vi "terminatePassPlay.vi"(8 "error in (no error)":errorcluster, 11 "Game in":refnum<class "Game.lvclass">) -> (0 "error out":errorcluster, 2 "terminate":bool, 3 "Game out":refnum<class "Game.lvclass">)   [LabVIEW 2018, in "Game.lvclass"]
uses:
  Game.lvclass
  Game.lvclass/Game.ctl
  Events_class/Events.lvclass/Events.ctl
  Read EventsRef.vi
  Events_class/Read ball_out.vi
  Events_class/Read touch.vi
  Events_class/Read id_touch.vi
  Events_class/Events.lvclass
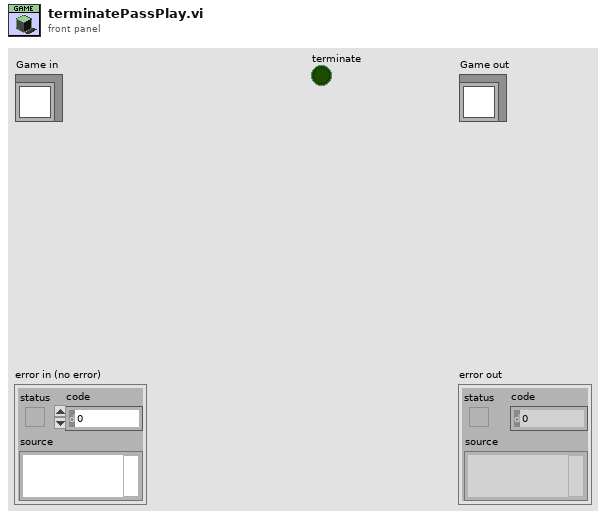
[diagram p1: front panel]
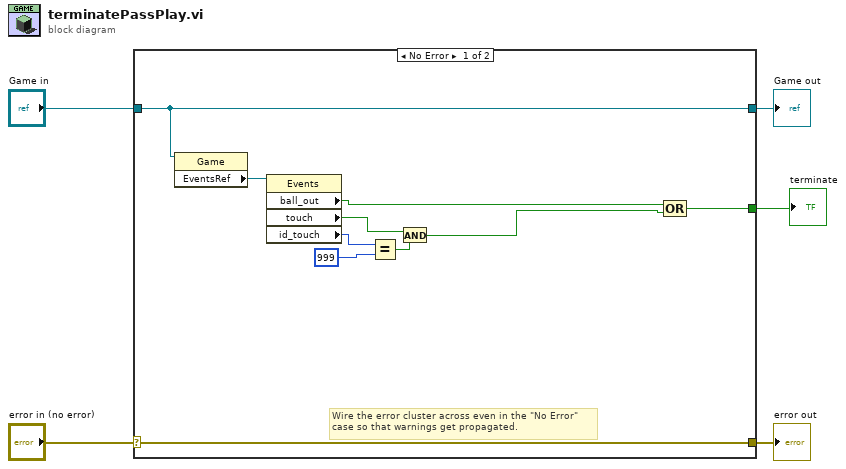
[diagram p0: block diagram]
diagram:
  n1 = case shown="No Error" "error in (no error)" {
    selector: "error in (no error)" -> [w15 w17]
    tunnel: [w15 w17] -> w4
    tunnel: [w14 w16] -> w2
    tunnel: "Game in" -> [w14 w16]
    tunnel: [w6 _] -> w1
    frame No Error {
      # "Wire the error cluster across even in the \"No Error\"\ncase so that warnings get propagated."
      n2 = property class="Game"(reference=w14) -> ("EventsRef"=w13:refnum<class "Events.lvclass">)  [unwired: 1 in, 2 out]
      n3 = property class="Events"(reference=w13) -> ("ball_out"=w12:bool, "touch"=w11:bool, "id_touch"=w9:i32)  [unwired: 1 in, 2 out]
      n4 = Equal?(x=w9, y=999) -> (x = y?=w10:bool)
      n5 = And(x=w11, y=w10) -> (x .and. y?=w7:bool)
      n6 = Compound Arithmetic op=OR(w12, w7) -> (w6:bool)
    }
    frame Error {
    }
  }
  "error out" <- w4
  "Game out" <- w2
  "terminate" <- w1
